vi "RM.getAllServerInfo.vi"(8 "error in":errorcluster, 11 "Item Ref in":T2 format="%.0x") -> (0 "error out":errorcluster, 2 "ServerInfo Array":T1[](array[typedef]) {"cd node ref" format="%.0x"}, 3 "Item Ref out":T2 format="%.0x")   [LabVIEW 2016, in "FPGA Resource Manager.lvlib"]
uses:
  FPGA Resource Manager.lvlib
  <vilib>/NI Veristand/Custom Device API/Custom Device Item Ref.ctl
  RM.serverInfo.ctl
  <vilib>/NI Veristand/Custom Device API/Custom Device API.lvlib
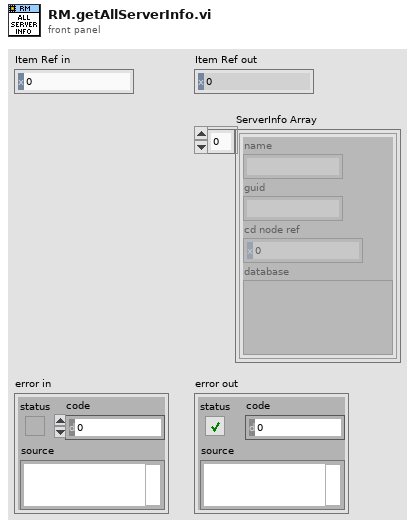
[diagram p1: front panel]
types:
  T1 = typedef "FPGA Resource Manager.lvlib/RM.serverInfo.ctl" = cluster{"name":string, "guid":string, "cd node ref":T2, "database":variant}
  T2 = typedef "Custom Device API.lvlib/Custom Device Item Ref.ctl" = u64
  T3 = typedef "Custom Device API.lvlib/Custom Device Item Info.ctl" = cluster{"Name":string, "Is Channel":bool, "GUID":string, "Is Waveform":bool}
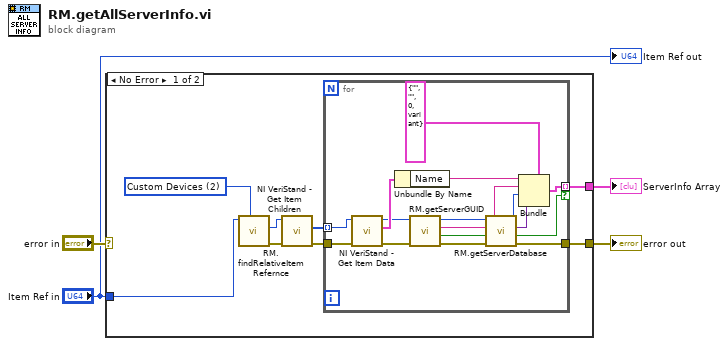
[diagram p0: block diagram]
diagram:
  n1 = case shown="No Error" "error in" {
    selector: "error in" -> [_ w28]
    tunnel: "Item Ref in" -> [w10 _]
    tunnel: [w12 w28] -> w3
    tunnel: [w6 _] -> w1
    frame No Error {
      w11 = u16 2 items=["Targets", "Controller", "Custom Devices", "This CD", "This CD/Group", "This CD/Group/SubGroup"] ("Relative Type")
      n2 = call "RM.findRelativeItemRefernce.vi"("Relative Type"=w11, "Item Ref in"=w10) -> ("error out"=w9:errorcluster, "Relative Item Ref Out"=w8:T2)  [unwired: 5 in, 3 out]
      n3 = call <vilib>:"NI VeriStand - Get Item Children.vi"("error in (no error)"=w9, "Item Ref in"=w8) -> ("error out"=w5:errorcluster, "Child Refs"=w7:T2[])  [unwired: 6 in, 2 out]
      n4 = for {
        tunnel: [w16] -> w12
        tunnel: w7 -> [w27] mode=indexing
        tunnel: [w22] -> w6 mode=indexing if=w17
        tunnel: w5 -> [w25]
        n5 = call <vilib>:"NI VeriStand - Get Item Data.vi"("error in (no error)"=w25, "Item Ref in"=w27) -> ("error out"=w21:errorcluster, "Item Info"=w26:T3, "Item Ref out"=w19:T2)  [unwired: 6 in, 1 out]
        n6 = Unbundle By Name(w26) -> ("Name"=w24:string)
        n7 = call "RM.getServerGUID.vi"("error in (no error)"=w21, "Item Ref in"=w19) -> ("error out"=w20:errorcluster, "Found?"=w17:bool, "ServerGUID"=w18:string, "Item Ref out"=w15:T2)  [unwired: 6 in]
        n8 = call "RM.getServerDatabase.vi"("error in (no error)"=w20, "Item Ref in"=w15) -> ("error out"=w16:errorcluster, "ServerDatabase"=w13:variant, "Item Ref out"=w14:T2)  [unwired: 6 in, 1 out]
        n9 = Bundle(cluster=T1 {"name"="", "guid"="", "cd node ref"=0, "database"=variant} ("serverInfo"), "name"=w24, "guid"=w18, "cd node ref"=w14, "database"=w13) -> (w22:T1)
      }
    }
    frame Error {
    }
  }
  "error out" <- w3
  "ServerInfo Array" <- w1
  "Item Ref out" <- "Item Ref in"
